vi "Stop Core.vi"(10 "final error code":i32, 11 "Nested in":refnum<class "MSS Remote Actor.lvclass">) -> (3 "Nested out":refnum<class "MSS Remote Actor.lvclass">)   [LabVIEW 2023, in "MSS Remote Actor.lvlib" / "MSS Remote Actor.lvclass"]
doc: "(<B>Filename</B>: Actor Framework.lvlib:Actor.lvclass:Stop Core.vi)\n\nDefines what the actor does before it stops. Use the <B>final error code</B> input to determine whether the actor shut down in response to an error.\n\nBy default, this method does nothing. A descendant class may override it to define behavior, such as shutting down any processes the actor initiated in its override of the Actor Core method."
uses:
  MSS Remote Actor.lvclass
  MSS Remote Actor.lvclass/MSS Remote Actor.ctl
  <vilib>/ActorFramework/Actor/Actor.lvclass
  HAL GOOP4/Measure and Stimulus Subsystems/Measure and Stimulus Subsystems.lvclass
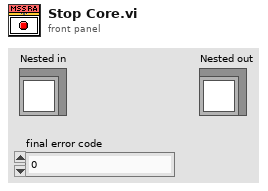
[diagram p1: front panel]
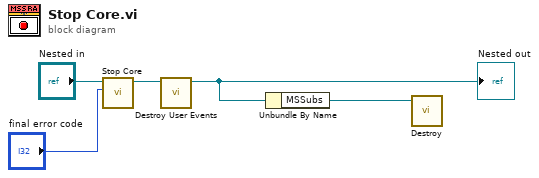
[diagram p0: block diagram]
diagram:
  n1 = call-parent "Stop Core.vi"("final error code"="final error code", "Actor in"="Nested in") -> ("Actor out"=w3:refnum<class "MSS Remote Actor.lvclass">)  [unwired: 9 in]
  n2 = call "Destroy User Events.vi"("UI Template in"=w3) -> ("UI Template out"=w2:refnum<class "MSS Remote Actor.lvclass">)  [unwired: 10 in]
  "Nested out" <- w2
  n3 = Unbundle By Name(w2) -> ("MSSubs"=w1:refnum<class "Measure and Stimulus Subsystems.lvclass">)
  n4 = call-dynamic "Destroy.vi"("reference in"=w1) -> ()  [unwired: 9 in, 2 out]
